vi "Analysis.LevelTransition.OPH.vi"(9 "Array in":dbl[][](array[numeric]), 10 "LVTransitionParameters":T1, 11 "Numeric":dbl) -> (3 "Array out":bool[](array[boolean]))   [LabVIEW 2014, in "NIAnalysis.lvlib"]
uses:
  NIAnalysis.lvlib
  Types/Public.LVAnalysis.ctl
  Types/Public.ChLVAnalysis.ctl
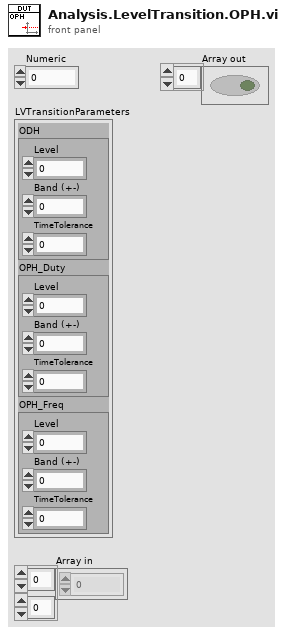
[diagram p1: front panel]
types:
  T1 = typedef "NIAnalysis.lvlib/Public.LVAnalysis.ctl" = cluster{"ODH":T2, "OPH_Duty":T2, "OPH_Freq":T2}
  T2 = typedef "NIAnalysis.lvlib/Public.ChLVAnalysis.ctl" = cluster{"Level":dbl, "Band (+-)":dbl, "TimeTolerance":dbl}
  T3 = cluster{"Scale":dbl, "Hi":dbl, "Lo":dbl, "dt":dbl, "Timeout":dbl}
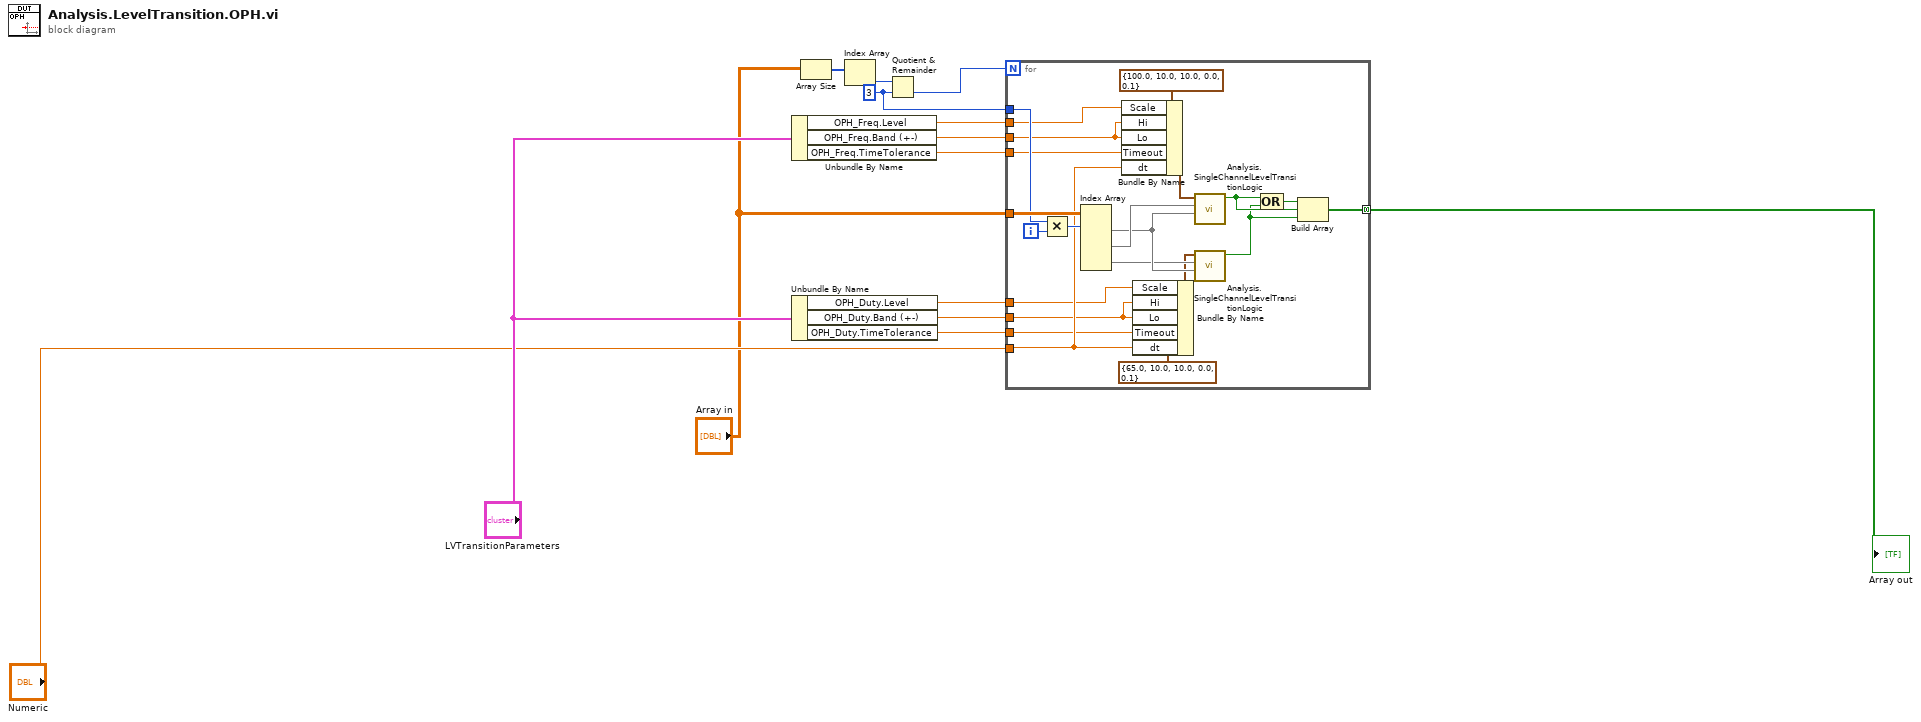
[diagram p0: block diagram]
diagram:
  w1 = 3 ("y")
  n1 = Unbundle By Name("LVTransitionParameters") -> ("OPH_Freq.Level"=w10:dbl, "OPH_Freq.Band (+-)"=w9:dbl, "OPH_Freq.TimeTolerance"=w8:dbl)
  n2 = Unbundle By Name("LVTransitionParameters") -> ("OPH_Duty.Level"=w13:dbl, "OPH_Duty.Band (+-)"=w12:dbl, "OPH_Duty.TimeTolerance"=w11:dbl)
  n3 = Array Size(array="Array in") -> (size(s)=w4:i32[])
  n4 = Index Array(array=w4) -> (element=w3:i32)  [unwired: 1 in]
  n5 = Quotient & Remainder(x=w3, y=w1) -> (floor(x/y)=w2:i32)  [unwired: 1 out]
  n6 = for {
    N: w2 -> [_]
    tunnel: "Array in" -> [w36]
    tunnel: w1 -> [w31]
    tunnel: [w30] -> w6 mode=concatenating
    tunnel: "Numeric" -> [w21]
    tunnel: w8 -> [w20]
    tunnel: w9 -> [w19]
    tunnel: w10 -> [w18]
    tunnel: w11 -> [w17]
    tunnel: w12 -> [w16]
    tunnel: w13 -> [w15]
    i -> [w33]
    n7 = Multiply(x=w31, y=w33) -> (x*y=w32:i32)
    n8 = Index Array(array=w36, index (row) #1=w32) -> (element #1=w29:dbl[], element #2=w34:dbl[], element #3=w28:dbl[])  [unwired: 5 in]
    n9 = Bundle By Name(cluster=T3 {"Scale"=100.0, "Hi"=10.0, "Lo"=10.0, "dt"=0.0, "Timeout"=0.1} ("Parameters"), "Scale"=w18, "Hi"=w19, "Lo"=w19, "Timeout"=w20, "dt"=w21) -> (w35:T3)
    n10 = Bundle By Name(cluster=T3 {"Scale"=65.0, "Hi"=10.0, "Lo"=10.0, "dt"=0.0, "Timeout"=0.1} ("Parameters"), "Scale"=w15, "Hi"=w16, "Lo"=w16, "Timeout"=w17, "dt"=w21) -> (w26:T3)
    n11 = call "Analysis.SingleChannelLevelTransitionLogic.vi"("Stimulus"=w29, "Response"=w34, "Parameters"=w35) -> ("Fail"=w24:bool)  [unwired: 8 in]
    n12 = call "Analysis.SingleChannelLevelTransitionLogic.vi"("Stimulus"=w29, "Response"=w28, "Parameters"=w26) -> ("Fail"=w23:bool)  [unwired: 8 in]
    n13 = Compound Arithmetic op=OR(w24, w23) -> (w22:bool)
    n14 = Build Array(w22, w24, w23) -> (w30:bool[])
  }
  "Array out" <- w6
